vi "Manual or Auto Control.vi"(8 "error in (no error)":errorcluster, 10 "Controller State":enum16{"Manual", "Auto"}(ring), 11 "Range Controller Actor in":refnum<class "Range Controller Actor.lvclass">) -> (0 "error out":errorcluster, 3 "Range Controller Actor out":refnum<class "Range Controller Actor.lvclass">)   [LabVIEW 2018, in "Range Controller.lvlib" / "Range Controller Actor.lvclass"]
uses:
  Range Controller Actor.lvclass
  Range Controller Actor.lvclass/Range Controller Actor.ctl
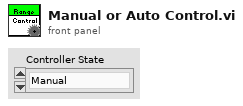
[diagram p1: front panel]
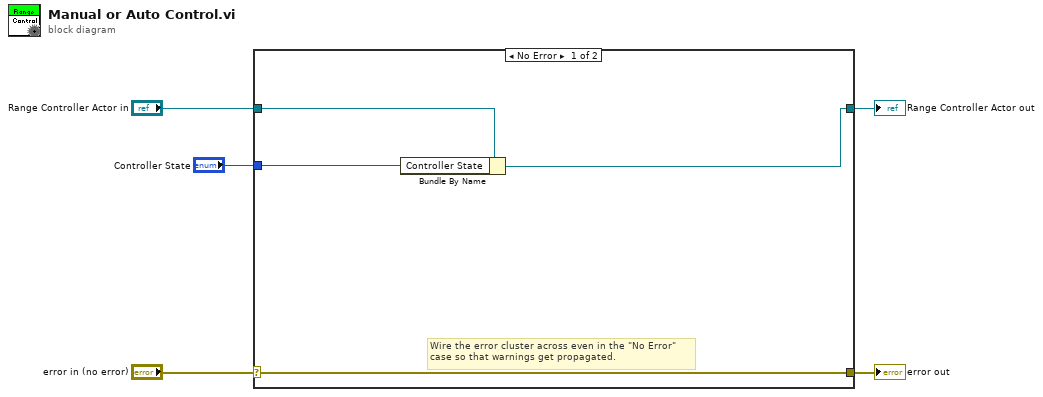
[diagram p0: block diagram]
diagram:
  n1 = case shown="No Error" "error in (no error)" {
    selector: "error in (no error)" -> [w9 w11]
    tunnel: [w9 w11] -> w4
    tunnel: [w6 w10] -> w2
    tunnel: "Range Controller Actor in" -> [w8 w10]
    tunnel: "Controller State" -> [w7 _]
    frame No Error {
      # "Wire the error cluster across even in the \"No Error\"\ncase so that warnings get propagated."
      n2 = Bundle By Name(cluster=w8, "Controller State"=w7) -> (w6:refnum<class "Range Controller Actor.lvclass">)
    }
    frame Error {
    }
  }
  "error out" <- w4
  "Range Controller Actor out" <- w2
